vi "Ping computer 2.vi"(7 "Ping Command (ping -n 1 -w 5)":string="ping -n 1 -w 5", 8 "error in":errorcluster, 11 "IP Address":string) -> (0 "error out":errorcluster, 1 "return code":i32, 2 "standard error":string, 3 "Ping Output":string, 4 "ping time [ms]":u32)   [LabVIEW 2013]
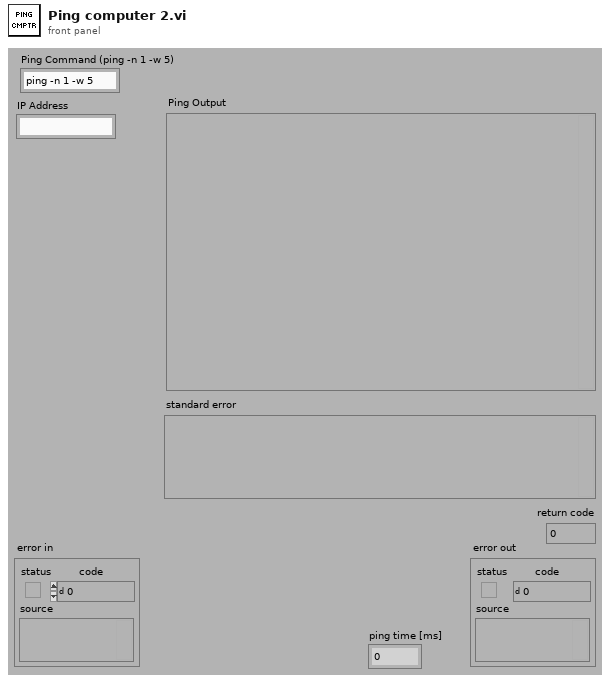
[diagram p1: front panel]
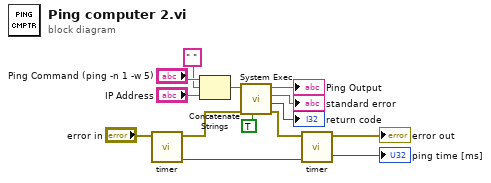
[diagram p0: block diagram]
diagram:
  n1 = call "timer.vi"("error in (no error)"="error in") -> ("time out [ms]"=w4:u32, "error out"=w7:errorcluster)  [unwired: 8 in, 1 out]
  n2 = Concatenate Strings("Ping Command (ping -n 1 -w 5)", " " ("string"), "IP Address") -> (w13:string)
  n3 = call <vilib>:"System Exec.vi"("run minimized? (F)"=TRUE, "error in (no error)"=w7, "command line"=w13) -> ("error out"=w6:errorcluster, "return code"=→"return code":i32, "standard error"=→"standard error":string, "standard output"=→"Ping Output":string)  [unwired: 3 in, 2 out]
  n4 = call "timer.vi"("time in [ms]"=w4, "error in (no error)"=w6) -> ("error out"=→"error out":errorcluster, "time difference [ms]"=→"ping time [ms]":u32)  [unwired: 8 out]
